vi "PullOutData.vi"(1 "WhichInd":i32, 2 "InputArray":i16[][](array[numeric])) -> (0 "OutVec":i16[](array[numeric]))   [LabVIEW 2018]
uses:
  D:/LabVIEW/LabVIEWProjects/dlcTAF/dlcTAF1.1/SubVIs/64bitC_code/PullOutData_C/bin/Debug/PullOutData_C.dll
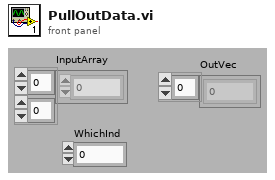
[diagram p1: front panel]
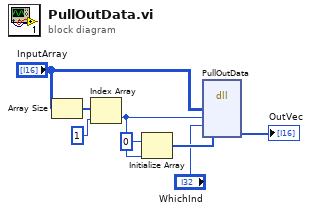
[diagram p0: block diagram]
diagram:
  n1 = Array Size(array="InputArray") -> (size(s)=w6:i32[])
  n2 = Index Array(array=w6, index=1) -> (element=w3:i32)
  n3 = Initialize Array(i16 0 ("element"), w3) -> (w2:i16[])
  n4 = dll-call lib="D:/LabVIEW/LabVIEWProjects/dlcTAF/dlcTAF1.1/SubVIs/64bitC_code/PullOutData_C/bin/Debug/PullOutData_C.dll" fn="PullOutData"("InputArray"="InputArray", "Ndat"=w3, "WhichInd"="WhichInd", "OutVec"=w2) -> ("OutVec"=→"OutVec":i16[])  [unwired: 7 in, 2 out]
